vi "KGN Get Concentrations.vi"(7 "scaling":dbl=1000000.0, 8 "Fehler (Eingang, kein Fehler)":errorcluster, 9 "Info Cluster":T1, 10 "VISA-Ressourcenname":refnum<visa-resource-name>, 11 "device (Eingang)":u32) -> (0 "Fehler (Ausgang)":errorcluster, 1 "Info Cluster out":T1, 2 "VISA-Ressourcenname out":refnum<visa-resource-name>, 3 "dup device (Ausgang)":u32, 4 "Input Concentrations (Ausgang)":T2(array[cluster]), 6 "Kommandos gesendet":string)   [LabVIEW 2020, in "Linearisierung v2.lvlib" / "Gasteiler.lvlib" / "HovaCAL_Interface.lvlib" / "KGN.lvlib" / "KGN GUI Get.lvlib"]
uses:
  KGN GUI Get.lvlib
  Controls/Info Cluster.ctl
  get/get.lvlib
  Controls/Controls.lvlib
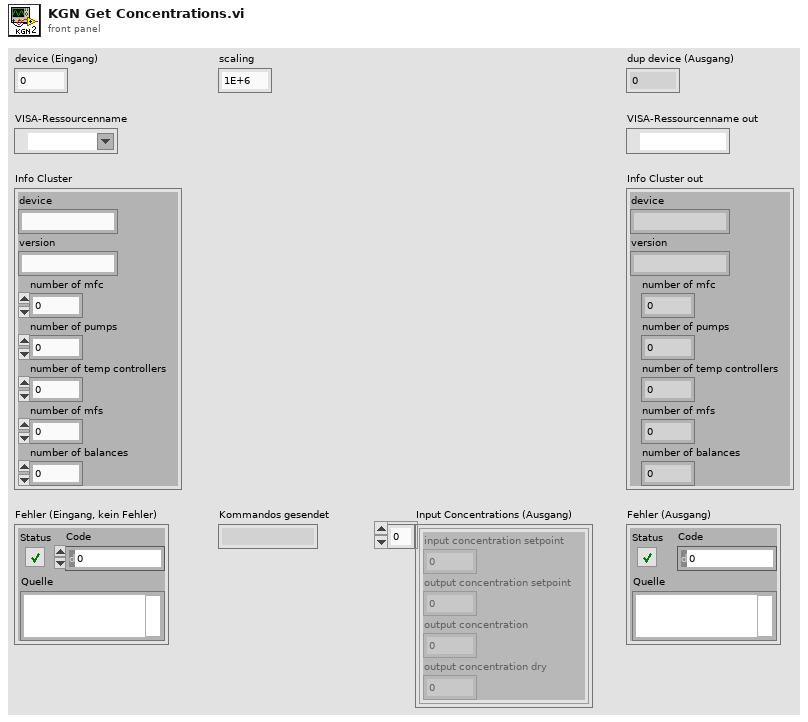
[diagram p1: front panel]
types:
  T1 = typedef "Linearisierung v2.lvlib/Gasteiler.lvlib/HovaCAL_Interface.lvlib/Controls.lvlib/Info Cluster.ctl" = cluster{"device":string, "version":string, "number of mfc":i32, "number of pumps":i32, "number of temp controllers":i32, "number of mfs":i32, "number of balances":i32}
  T2 = cluster{"input concentration setpoint":dbl, "output concentration setpoint":dbl, "output concentration":dbl, "output concentration dry":dbl}[]
  T3 = cluster{"input concentration setpoint":dbl, "output concentration setpoint":dbl, "output concentration":dbl, "output concentration dry":dbl}
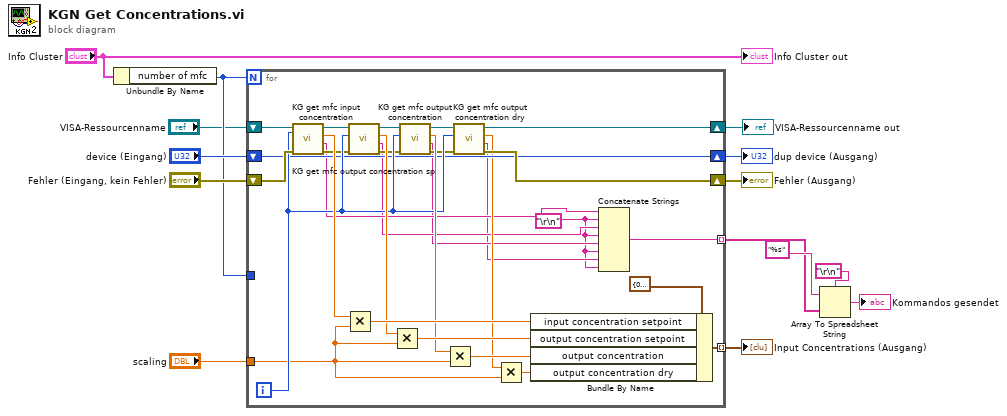
[diagram p0: block diagram]
diagram:
  n1 = Unbundle By Name("Info Cluster") -> ("number of mfc"=w8:i32)
  n2 = for {
    N: w8 -> [_]
    tunnel: "scaling" -> [w29]
    tunnel: w8 -> [_]
    tunnel: [w38] -> w7 mode=indexing
    shift-right: [w34] -> w12
    shift-left: "Fehler (Eingang, kein Fehler)" -> [w36]
    shift-right: [w33] -> w13
    shift-left: "device (Eingang)" -> [w33]
    shift-right: [w27] -> w5
    shift-left: "VISA-Ressourcenname" -> [w28]
    tunnel: [w15] -> w2 mode=indexing
    i -> [w35]
    w16 = "\r\n"
    n3 = call "KG get mfc input concentration.vi"("Fehler (Eingang, kein Fehler)"=w36, "mfc"=w35, "VISA-Ressourcenname"=w28) -> ("Fehler (Ausgang)"=w25:errorcluster, "Kommando gesendet"=w20:string, "concentration"=w37:dbl, "VISA-Ressourcenname (Ausgang)"=w26:refnum<visa-resource-name>)  [unwired: 5 in]
    n4 = Multiply(x=w37, y=w29) -> (x*y=w41:dbl)
    n5 = call "KG get mfc output concentration sp.vi"("Fehler (Eingang, kein Fehler)"=w25, "mfc"=w35, "VISA-Ressourcenname"=w26) -> ("Fehler (Ausgang)"=w24:errorcluster, "Kommando gesendet"=w19:string, "concentration"=w39:dbl, "VISA-Ressourcenname (Ausgang)"=w22:refnum<visa-resource-name>)  [unwired: 5 in]
    n6 = Multiply(x=w39, y=w29) -> (x*y=w42:dbl)
    n7 = call "KG get mfc output concentration.vi"("Fehler (Eingang, kein Fehler)"=w24, "mfc"=w35, "VISA-Ressourcenname"=w22) -> ("Fehler (Ausgang)"=w23:errorcluster, "Kommando gesendet"=w18:string, "concentration"=w40:dbl, "VISA-Ressourcenname (Ausgang)"=w21:refnum<visa-resource-name>)  [unwired: 5 in]
    n8 = Multiply(x=w40, y=w29) -> (x*y=w43:dbl)
    n9 = call "KG get mfc output concentration dry.vi"("Fehler (Eingang, kein Fehler)"=w23, "mfc"=w35, "VISA-Ressourcenname"=w21) -> ("Fehler (Ausgang)"=w34:errorcluster, "Kokmando gesendet"=w17:string, "concentration"=w30:dbl, "VISA-Ressourcenname (Ausgang)"=w27:refnum<visa-resource-name>)  [unwired: 5 in]
    n10 = Multiply(x=w30, y=w29) -> (x*y=w31:dbl)
    n11 = Bundle By Name(cluster=T3 {"input concentration setpoint"=0.0, "output concentration setpoint"=0.0, "output concentration"=0.0, "output concentration dry"=0.0} ("Actual Values Cluster"), "input concentration setpoint"=w41, "output concentration setpoint"=w42, "output concentration"=w43, "output concentration dry"=w31) -> (w38:T3)
    n12 = Concatenate Strings(w20, w16, w19, w16, w18, w16, w17, w16) -> (w15:string)
  }
  "Input Concentrations (Ausgang)" <- w7
  "dup device (Ausgang)" <- w13
  "Fehler (Ausgang)" <- w12
  "VISA-Ressourcenname out" <- w5
  n13 = Array To Spreadsheet String(delimiter (Tab)="\r\n", array=w2, 3:"%s" ("Format-String")) -> (spreadsheet string=→"Kommandos gesendet":string)
  "Info Cluster out" <- "Info Cluster"
